vi "rs3_RGB_to_Picture5.vi"(0 "RGB array":u8[](array[numeric]), 1 "Color format":enum16{"Monochrome", "RGB internal (RGB)"}(ring), 5 "RGB  X, width":i32, 7 "RGB Y, height":i32, 9 "AWB":bool, 11 "error in (no error)":errorcluster, 12 "White Balance":T1={"Red"=1.0, "Green"=1.0, "Blue"=1.0, "Gain"=1.0} {"Gain" format="%_3g"; "Blue" format="%_3g"; "Green" format="%_3g"; "Red" format="%_3g"}, 14 "White Balance":bool) -> (6 "new picture":picture, 15 "error out":errorcluster)   [LabVIEW 2017, in "libRealSense3.lvlib"]
doc: "This converts an 1D input array into a 2D picture, and applies some white balance correction if requested."
uses:
  <vilib>/Analysis/baseanly.llb/Mean (DBL).vi
  libRealSense3.lvlib
  <vilib>/Analysis/NI_AALBase.lvlib
panel:
  # "RS3 RGB to Picture 5"
  # "(C) Intel Corp. 2017,  AGJ"
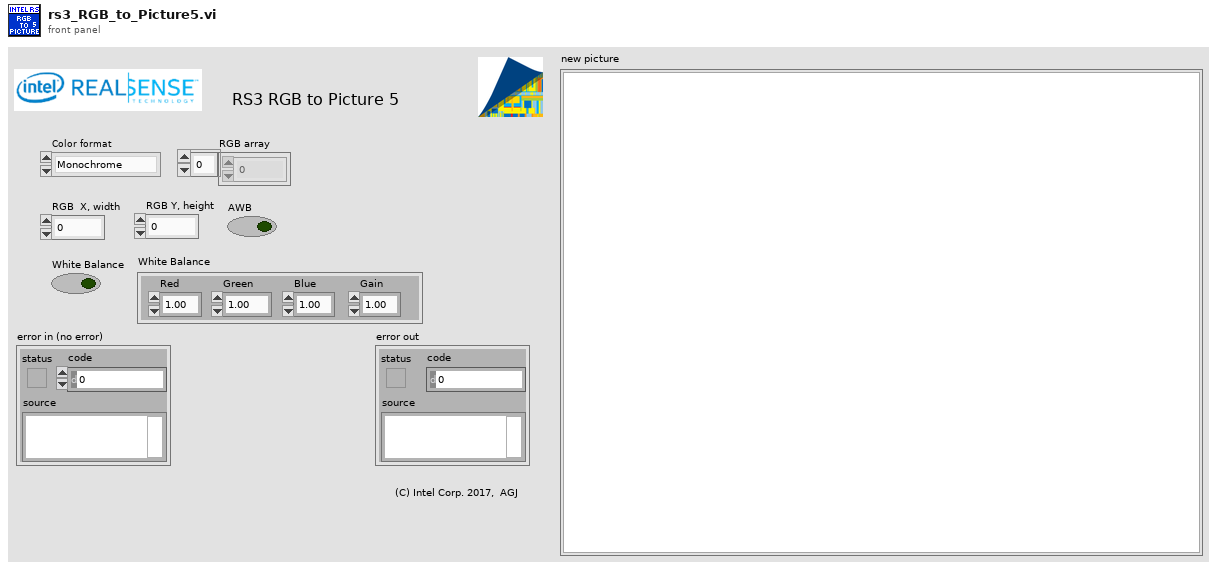
[diagram p1: front panel]
types:
  T1 = cluster{"Red":dbl, "Green":dbl, "Blue":dbl, "Gain":dbl}
  T2 = typedef "imagedata.ctl" = cluster{"image type":i32, "image depth":i32, "image":u8[], "mask":u8[], "colors":u32[], "Rectangle":cluster{"left":i16, "top":i16, "right":i16, "bottom":i16}}
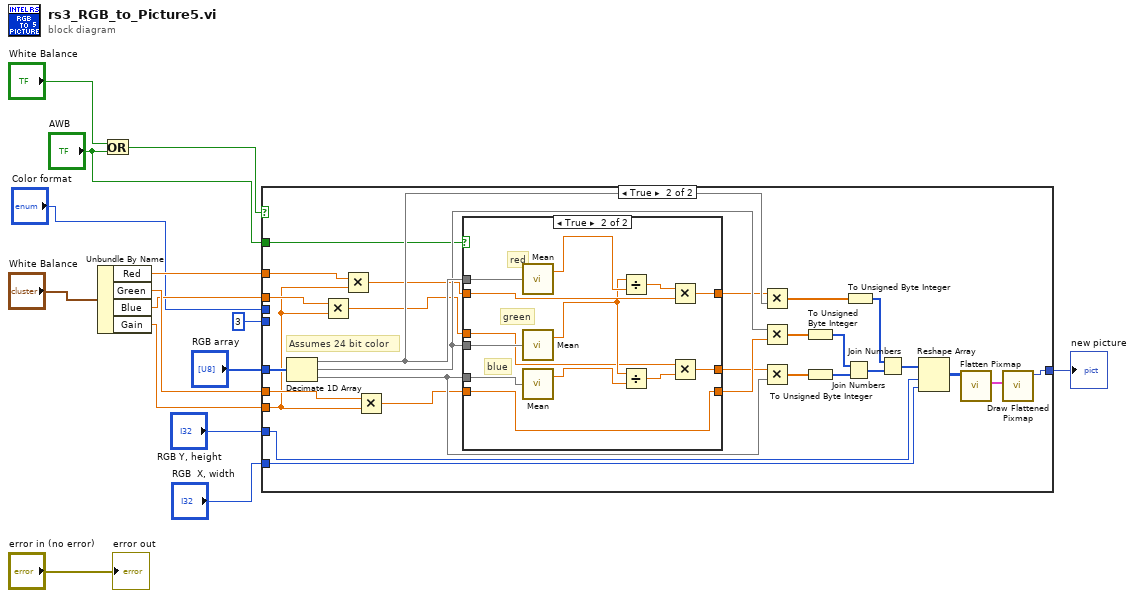
[diagram p0: block diagram]
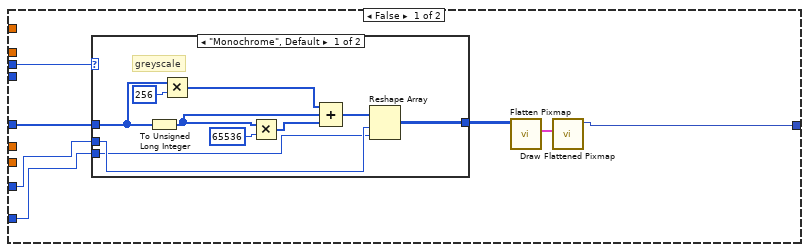
[diagram p2: hidden frame]
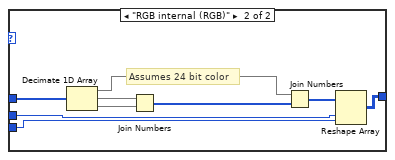
[diagram p3: hidden frame]
diagram:
  n1 = Unbundle By Name("White Balance") -> ("Red"=w10:dbl, "Green"=w9:dbl, "Blue"=w8:dbl, "Gain"=w1:dbl)
  n2 = Or(x="White Balance", y="AWB") -> (x .or. y?=w3:bool)
  n3 = case shown="True" w3 {
    tunnel: [w22 w57] -> w15
    tunnel: "RGB array" -> [w21 w65]
    tunnel: "RGB Y, height" -> [w20 w56]
    tunnel: "RGB  X, width" -> [w19 w64]
    tunnel: 3 ("# of bytes/number") -> [_ _]
    tunnel: w10 -> [_ w48]
    tunnel: w9 -> [_ w46]
    tunnel: w8 -> [_ w44]
    tunnel: "AWB" -> [_ w49]
    tunnel: "Color format" -> [w18 _]
    tunnel: w1 -> [_ w42]
    frame False {
      n4 = case shown="\"Monochrome\", Default" w18 {
        tunnel: [w30 w40] -> w17
        tunnel: w21 -> [w26 w38]
        tunnel: w20 -> [w32 w37]
        tunnel: w19 -> [w31 w36]
        frame "Monochrome", Default {
          # "greyscale"
          n5 = To Unsigned Long Integer(number=w26) -> (unsigned 32bit integer=w23:u32[])
          n6 = Multiply(x=w26, y=u32 256) -> (x*y=w27:u32[])
          n7 = Multiply(x=w23, y=u32 65536) -> (x*y=w25:u32[])
          n8 = Compound Arithmetic op=ADD(w27, w23, w25) -> (w24:u32[])
          n9 = Reshape Array(w24, w32, w31) -> (w30:u32[][])
        }
        frame "RGB internal (RGB)" {
          # "Assumes 24 bit color"
          n10 = Decimate 1D Array(w38) -> (w35:u8[], w34:u8[], w33:u8[])
          n11 = Join Numbers(hi=w34, lo=w33) -> ((hi.lo)=w41:u16[])
          n12 = Join Numbers(hi=w35, lo=w41) -> ((hi.lo)=w39:u32[])
          n13 = Reshape Array(w39, w37, w36) -> (w40:u32[][])
        }
      }
      n14 = call <vilib>:"Flatten Pixmap.vi"("24-bit pixmap"=w17) -> ("image data"=w16:T2)  [unwired: 10 in]
      n15 = call <vilib>:"Draw Flattened Pixmap.vi"("image data"=w16) -> ("new picture"=w22:picture)  [unwired: 8 in]
    }
    frame True {
      # "Assumes 24 bit color"
      n16 = Decimate 1D Array(w65) -> (w55:u8[], w54:u8[], w53:u8[])
      n17 = Multiply(x=w44, y=w42) -> (x*y=w43:dbl)
      n18 = Multiply(x=w48, y=w42) -> (x*y=w47:dbl)
      n19 = Multiply(x=w46, y=w42) -> (x*y=w45:dbl)
      n20 = case shown="True" w49 {
        tunnel: w55 -> [_ w85]
        tunnel: w54 -> [_ w84]
        tunnel: w53 -> [_ w83]
        tunnel: [w72 w78] -> w52
        tunnel: w47 -> [w72 w79]
        tunnel: [w71 w73] -> w51
        tunnel: w45 -> [w71 w73]
        tunnel: w43 -> [w70 w75]
        tunnel: [w70 w74] -> w50
        frame False {
        }
        frame True {
          # "blue"
          # "green"
          # "red"
          n21 = call-poly <vilib>:"Mean.vi"("X"=w85) -> ("mean"=w82:dbl)  [unwired: 1 out]
          n22 = call-poly <vilib>:"Mean.vi"("X"=w84) -> ("mean"=w77:dbl)  [unwired: 1 out]
          n23 = call-poly <vilib>:"Mean.vi"("X"=w83) -> ("mean"=w81:dbl)  [unwired: 1 out]
          n24 = Divide(x=w77, y=w82) -> (x/y=w80:dbl)
          n25 = Divide(x=w77, y=w81) -> (x/y=w76:dbl)
          n26 = Multiply(x=w80, y=w79) -> (x*y=w78:dbl)
          n27 = Multiply(x=w75, y=w76) -> (x*y=w74:dbl)
        }
      }
      n28 = Multiply(x=w52, y=w55) -> (x*y=w63:dbl[])
      n29 = Multiply(x=w54, y=w51) -> (x*y=w59:dbl[])
      n30 = Multiply(x=w50, y=w53) -> (x*y=w60:dbl[])
      n31 = To Unsigned Byte Integer(number=w59) -> (unsigned 8bit integer=w61:u8[])
      n32 = To Unsigned Byte Integer(number=w60) -> (unsigned 8bit integer=w58:u8[])
      n33 = Join Numbers(hi=w61, lo=w58) -> ((hi.lo)=w69:u16[])
      n34 = To Unsigned Byte Integer(number=w63) -> (unsigned 8bit integer=w62:u8[])
      n35 = Join Numbers(hi=w62, lo=w69) -> ((hi.lo)=w66:u32[])
      n36 = Reshape Array(w66, w56, w64) -> (w68:u32[][])
      n37 = call <vilib>:"Flatten Pixmap.vi"("24-bit pixmap"=w68) -> ("image data"=w67:T2)  [unwired: 10 in]
      n38 = call <vilib>:"Draw Flattened Pixmap.vi"("image data"=w67) -> ("new picture"=w57:picture)  [unwired: 8 in]
    }
  }
  "new picture" <- w15
  "error out" <- "error in (no error)"
